vi "Foot_GCP.vi"(0 "Gyro":sgl, 1 "High 검출값":sgl=400.0, 2 "Low 기준값":sgl=-400.0, 3 "MID 중간값":sgl=-200.0) -> (8 "Gait NUM":u32, 10 "GCP (%)":sgl format="%#.1f", 12 "Gait TIME (msec)":u32, 14 "HS":bool, 15 "FF":bool, 16 "TO":bool, 17 "SS":bool, 18 "MS":bool, 19 "SE":bool)   [LabVIEW 2019]
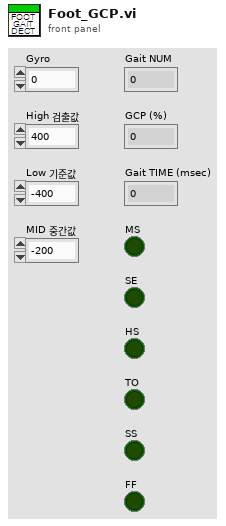
[diagram p1: front panel]
types:
  T1 = enum16{"Init", "MS", "SE", "HS", "FF", "TO", "SS"}
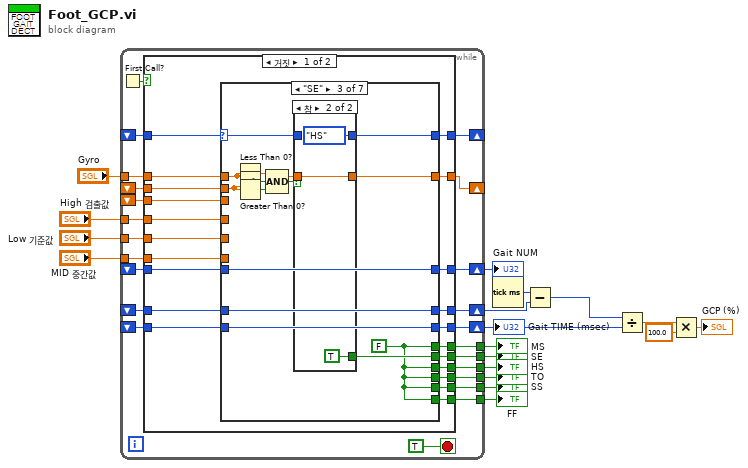
[diagram p0: block diagram]
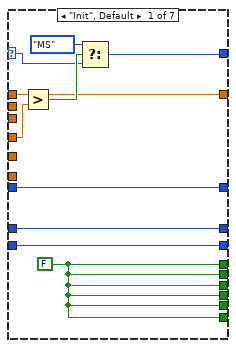
[diagram p2: hidden frame]
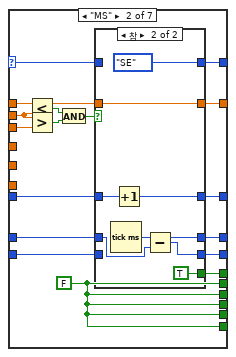
[diagram p3: hidden frame]
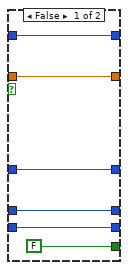
[diagram p4: hidden frame]
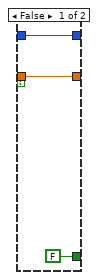
[diagram p5: hidden frame]
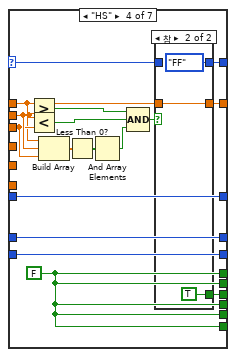
[diagram p6: hidden frame]
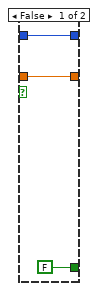
[diagram p7: hidden frame]
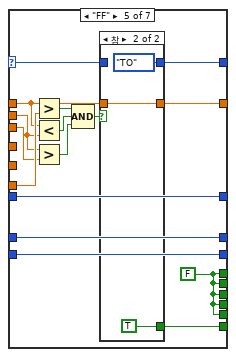
[diagram p8: hidden frame]
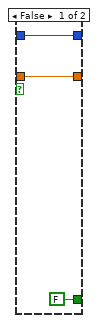
[diagram p9: hidden frame]
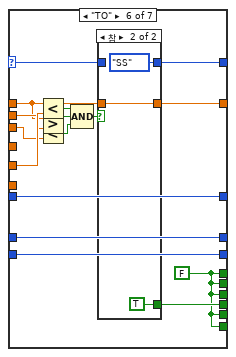
[diagram p10: hidden frame]
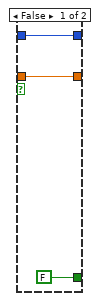
[diagram p11: hidden frame]
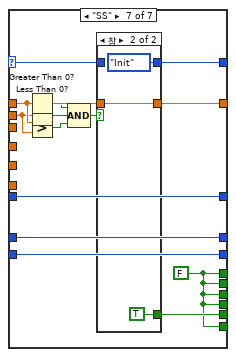
[diagram p12: hidden frame]
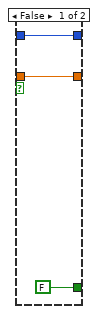
[diagram p13: hidden frame]
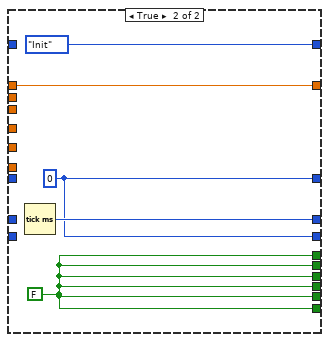
[diagram p14: hidden frame]
diagram:
  n1 = while {
    tunnel: "High 검출값" -> [w37]
    tunnel: "Low 기준값" -> [w25]
    shift-right: [w39] -> _
    shift-left: _ -> [w38]
    shift-right: [w27] -> _
    shift-left: _ -> [w36]
    shift-left: _ -> [w35]
    shift-right: [w34] -> w5
    shift-left: _ -> [w33]
    shift-right: [w32] -> w7
    shift-left: _ -> [w31]
    shift-right: [w30] -> w12
    shift-left: _ -> [w29]
    tunnel: [w28] -> w17
    tunnel: [w19] -> w18
    tunnel: [w26] -> w13
    tunnel: [w24] -> w15
    tunnel: "Gyro" -> [w23]
    tunnel: [w22] -> w16
    tunnel: "MID 중간값" -> [w21]
    tunnel: [w20] -> w14
    stop <- TRUE stop-if-true
    n2 = First Call?() -> (First Call?: T/F=w40:bool)
    n3 = case shown="거짓" w40 {
      tunnel: [w59 T1."Init"] -> w39
      tunnel: w38 -> [w62 _]
      tunnel: w23 -> [w61 w212]
      tunnel: w37 -> [w60 _]
      tunnel: w36 -> [w58 _]
      tunnel: w35 -> [w57 _]
      tunnel: [w56 w213] -> w34
      tunnel: w33 -> [w55 _]
      tunnel: [w54 w214] -> w32
      tunnel: w31 -> [w53 _]
      tunnel: [w52 w213] -> w30
      tunnel: w29 -> [w51 _]
      tunnel: [w50 w211] -> w28
      tunnel: [w49 w211] -> w19
      tunnel: [w48 w212] -> w27
      tunnel: [w47 w211] -> w26
      tunnel: w25 -> [w46 _]
      tunnel: [w45 w211] -> w24
      tunnel: [w44 w211] -> w22
      tunnel: w21 -> [w43 _]
      tunnel: [w42 w211] -> w20
      frame False {
        n4 = case shown="\"SE\"" w62 {
          selector: w62 -> [w70 w81 w117 w133 w162 w176 w202]
          tunnel: w61 -> [w65 w76 w110 w132 w158 w172 w204]
          tunnel: w60 -> [w72 _ _ _ _ _ _]
          tunnel: [w69 w84 w116 w134 w161 w177 w203] -> w59
          tunnel: w58 -> [_ w89 w109 w138 w157 w183 w201]
          tunnel: w57 -> [_ w88 _ w137 w156 w182 _]
          tunnel: [w68 w83 w115 w129 w151 w175 w196] -> w56
          tunnel: w55 -> [w68 w82 w115 w129 w151 w175 w196]
          tunnel: [w67 w80 w114 w128 w150 w174 w195] -> w54
          tunnel: w53 -> [w67 w79 w114 w128 w150 w174 w195]
          tunnel: [w66 w78 w113 w127 w149 w173 w194] -> w52
          tunnel: w51 -> [w66 w77 w113 w127 w149 w173 w194]
          tunnel: [w63 w74 w104 w124 w147 w169 w191] -> w50
          tunnel: [w63 w73 w112 w124 w147 w169 w191] -> w49
          tunnel: [w65 w75 w111 w130 w160 w171 w192] -> w48
          tunnel: [w63 w73 w104 w131 w147 w169 w191] -> w47
          tunnel: w46 -> [_ _ _ _ _ w184 _]
          tunnel: [w63 w73 w104 w124 w147 w170 w191] -> w45
          tunnel: [w63 w73 w104 w124 w147 w169 w193] -> w44
          tunnel: w43 -> [_ _ _ _ w159 _ _]
          tunnel: [w63 w73 w104 w124 w148 w169 w191] -> w42
          frame "Init", Default {
            w63 = FALSE
            n5 = Greater?(x=w65, y=w72) -> (0:w71:bool)
            n6 = Select(t=T1."MS", s=w71, f=w70) -> (s? t:f=w69:T1)
          }
          frame "MS" {
            w73 = FALSE
            n7 = Less?(x=w76, y=w89) -> (x < y?=w87:bool)
            n8 = Greater?(x=w89, y=w88) -> (0:w86:bool)
            n9 = And(x=w87, y=w86) -> (x .and. y?=w85:bool)
            n10 = case shown="참" w85 {
              tunnel: [w94 T1."SE"] -> w84
              tunnel: [w95 w103] -> w83
              tunnel: w82 -> [w95 w102]
              tunnel: w81 -> [w94 _]
              tunnel: [w93 w101] -> w80
              tunnel: w79 -> [w93 w100]
              tunnel: [w92 w99] -> w78
              tunnel: w77 -> [w92 _]
              tunnel: [w90 w98] -> w75
              tunnel: w76 -> [w90 w98]
              tunnel: [FALSE TRUE] -> w74
              frame False {
              }
              frame True {
                n11 = Tick Count (ms)() -> (millisecond timer value=w101:u32)
                n12 = Increment(x=w102) -> (x+1=w103:u32)
                n13 = Subtract(x=w101, y=w100) -> (x-y=w99:u32)
              }
            }
          }
          frame "SE" {
            w104 = FALSE
            n14 = Less Than 0?(x=w110) -> (x < 0?=w108:bool)
            n15 = Less?(x=w110, y=w109) -> (x < y?=w107:bool)
            n16 = Greater Than 0?(x=w109) -> (x > 0?=w106:bool)
            n17 = Compound Arithmetic op=AND ("복합 연산")(w108, w107, w106) -> (w105:bool)
            n18 = case shown="참" w105 {
              tunnel: w117 -> [w120 _]
              tunnel: [w120 T1."HS"] -> w116
              tunnel: [FALSE TRUE] -> w112
              tunnel: w110 -> [w118 w123]
              tunnel: [w118 w123] -> w111
              frame False {
              }
              frame True {
              }
            }
          }
          frame "HS" {
            w124 = FALSE
            n19 = Greater?(x=w132, y=w138) -> (0:w140:bool)
            n20 = Less?(x=w138, y=w137) -> (x < y?=w139:bool)
            n21 = Build Array(w132, w138, w137) -> (w136:sgl[])
            n22 = Less Than 0?(x=w136) -> (x < 0?=w135:bool[])
            n23 = And Array Elements(Boolean array=w135) -> (logical AND=w125:bool)
            n24 = Compound Arithmetic op=AND ("복합 연산")(w140, w139, w125) -> (w126:bool)
            n25 = case shown="참" w126 {
              tunnel: [w143 T1."FF"] -> w134
              tunnel: w133 -> [w143 _]
              tunnel: w132 -> [w141 w146]
              tunnel: [FALSE TRUE] -> w131
              tunnel: [w141 w146] -> w130
              frame False {
              }
              frame True {
              }
            }
          }
          frame "FF" {
            w147 = FALSE
            n26 = Greater?(x=w158, y=w159) -> (0:w155:bool)
            n27 = Less?(x=w158, y=w157) -> (x < y?=w154:bool)
            n28 = Greater?(x=w157, y=w156) -> (0:w153:bool)
            n29 = Compound Arithmetic op=AND ("복합 연산")(w155, w154, w153) -> (w152:bool)
            n30 = case shown="참" w152 {
              tunnel: w162 -> [w164 _]
              tunnel: [w164 T1."TO"] -> w161
              tunnel: [w165 w167] -> w160
              tunnel: w158 -> [w165 w167]
              tunnel: [FALSE TRUE] -> w148
              frame False {
              }
              frame True {
              }
            }
          }
          frame "TO" {
            w169 = FALSE
            n31 = Less?(x=w172, y=w184) -> (x < y?=w181:bool)
            n32 = Greater?(x=w172, y=w183) -> (0:w180:bool)
            n33 = Less?(x=w183, y=w182) -> (x < y?=w179:bool)
            n34 = Compound Arithmetic op=AND ("복합 연산")(w181, w180, w179) -> (w178:bool)
            n35 = case shown="참" w178 {
              tunnel: [w187 T1."SS"] -> w177
              tunnel: w176 -> [w187 _]
              tunnel: w172 -> [w186 w190]
              tunnel: [w186 w190] -> w171
              tunnel: [FALSE TRUE] -> w170
              frame False {
              }
              frame True {
              }
            }
          }
          frame "SS" {
            w191 = FALSE
            n36 = Greater Than 0?(x=w204) -> (x > 0?=w200:bool)
            n37 = Less Than 0?(x=w201) -> (x < 0?=w199:bool)
            n38 = Greater?(x=w204, y=w201) -> (0:w198:bool)
            n39 = Compound Arithmetic op=AND ("복합 연산")(w200, w199, w198) -> (w197:bool)
            n40 = case shown="참" w197 {
              tunnel: [w207 T1."Init"] -> w203
              tunnel: w202 -> [w207 _]
              tunnel: w204 -> [w206 w210]
              tunnel: [FALSE TRUE] -> w193
              tunnel: [w206 w210] -> w192
              frame False {
              }
              frame True {
              }
            }
          }
        }
      }
      frame True {
        w211 = FALSE
        w213 = u32 0
        n41 = Tick Count (ms)() -> (millisecond timer value=w214:u32)
      }
    }
  }
  "Gait NUM" <- w5
  "Gait TIME (msec)" <- w12
  "HS" <- w13
  "FF" <- w14
  "TO" <- w15
  "SS" <- w16
  "MS" <- w17
  "SE" <- w18
  n42 = Tick Count (ms)() -> (millisecond timer value=w6:u32)
  n43 = Subtract(x=w6, y=w7) -> (x-y=w11:u32)
  n44 = Divide ("나누기")(x=w11, y=w12) -> (x/y=w8:sgl)
  n45 = Multiply(x=w8, y=sgl 100.0) -> (x*y=→"GCP (%)":sgl)
